vi "Connector0 Analog Output.vi"(0 "Packets":u64[](array[numeric])=[0, 0]) -> ()   [LabVIEW 2010]
uses:
  <vilib>/eio/EIONode/EIONode.xnode
  <vilib>/rvi/eio/nirviEIOImplementation/nirviEIOImplementation.xnode
  <vilib>/rvi/eio/common/nirviEmuClasses.ctl
  <vilib>/rvi/eio/common/nirviEmuTemplateMethod_noerrors.vi
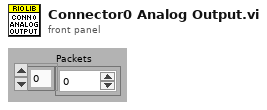
[diagram p1: front panel]
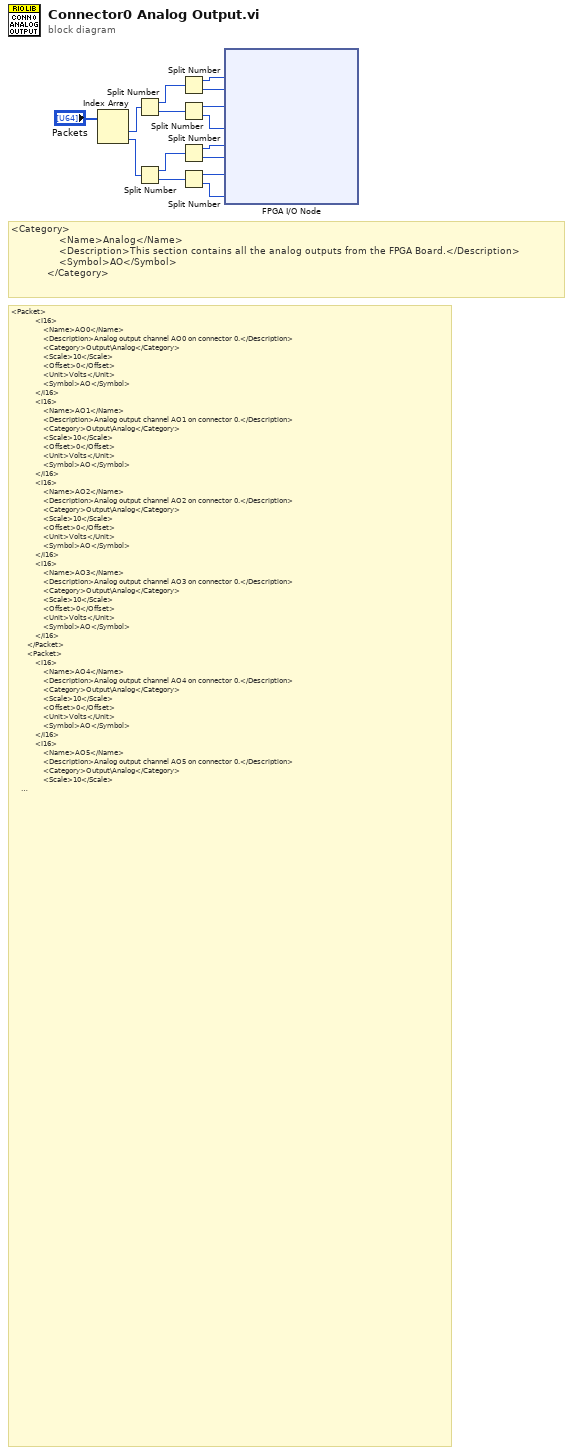
[diagram p0: block diagram]
diagram:
  # "<Category>\n                <Name>Analog</Name>\n                <Description>This section contains all the analog outputs from the FPGA Board.</Description>\n                <Symbol>AO</Symbol>\n            </Category>"
  # "<Packet>\n            <I16>\n                <Name>AO0</Name>\n                <Description>Analog output channel AO0 on connector 0.</Description>\n                <Category>Output\\Analog</Category>\n                <Scale>10</Scale>\n                <Offset>0</Offset>\n                <Unit>Volts</Unit>\n                <Symbol>AO</Symbol>\n            </I16>\n            <I16>\n                <Name>AO1</Name>\n                <Description>Analog output channel AO1 on connector 0.</Description>\n                <Category>Output\\Analog</Category>\n                <Scale>10</Scale>\n                <Offset>0</Offset>\n                <Unit>Volts</Unit>\n                <Symbol>AO</Symbol>\n            </I16>\n            <I16>\n                <Name>AO2</Name>\n                <Description>Analog output channel AO2 on connector 0.</Description>\n                <Category>Output\\Analog</Category>\n                <Scale>10</Scale>\n                <Offset>0</Offset>\n                <Unit>Volts</Unit>\n                <Symbol>AO</Symbol>\n            </I16>\n            <I16>\n                <Name>AO3</Name>\n                <Description>Analog output channel AO3 on connector 0.</Description>\n                <Category>Output\\Analog</Category>\n                <Scale>10</Scale>\n                <Offset>0</Offset>\n                <Unit>Volts</Unit>\n                <Symbol>AO</Symbol>\n            </I16>\n        </Packet>\n        <Packet>\n            <I16>\n                <Name>AO4</Name>\n                <Description>Analog output channel AO4 on connector 0.</Description>\n                <Category>Output\\Analog</Category>\n                <Scale>10</Scale>\n                <Offset>0</Offset>\n                <Unit>Volts</Unit>\n                <Symbol>AO</Symbol>\n            </I16>\n            <I16>\n                <Name>AO5</Name>\n                <Description>Analog output channel AO5 on connector 0.</Description>\n                <Category>Output\\Analog</Category>\n                <Scale>10</Scale>\n                <Offset>0</Offset>\n                <Unit>Volts</Unit>\n                <Symbol>AO</Symbol>\n            </I16>\n            <I16>\n                <Name>AO6</Name>\n                <Description>Analog output channel AO6 on connector 0.</Description>\n                <Category>Output\\Analog</Category>\n                <Scale>10</Scale>\n                <Offset>0</Offset>\n                <Unit>Volts</Unit>\n                <Symbol>AO</Symbol>\n            </I16>\n            <I16>\n                <Name>AO7</Name>\n                <Description>Analog output channel AO7 on connector 0.</Description>\n                <Category>Output\\Analog</Category>\n                <Scale>10</Scale>\n                <Offset>0</Offset>\n                <Unit>Volts</Unit>\n                <Symbol>AO</Symbol>\n            </I16>\n        </Packet>"
  n1 = Index Array(array="Packets") -> (element #1=w14:u64, element #2=w15:u64)  [unwired: 2 in]
  n2 = Split Number(x=w14) -> (hi(x)=w3:u32, lo(x)=w4:u32)
  n3 = Split Number(x=w15) -> (hi(x)=w2:u32, lo(x)=w1:u32)
  n4 = Split Number(x=w3) -> (hi(x)=w5:u16, lo(x)=w12:u16)
  n5 = Split Number(x=w4) -> (hi(x)=w11:u16, lo(x)=w10:u16)
  n6 = Split Number(x=w2) -> (hi(x)=w9:u16, lo(x)=w8:u16)
  n7 = Split Number(x=w1) -> (hi(x)=w7:u16, lo(x)=w6:u16)
  n8 = xnode "FPGA I/O Node"("Connector0/AO3"=w5, "Connector0/AO2"=w12, "Connector0/AO1"=w11, "Connector0/AO0"=w10, "Connector0/AO7"=w9, "Connector0/AO6"=w8, "Connector0/AO5"=w7, "Connector0/AO4"=w6) -> ()  [unwired: 8 in, 8 out]
